vi "шкала вакуума.vi"(11 "Vak_in":dbl) -> (0 "Vak_out_txt":string, 3 "Vak_out":dbl)   [LabVIEW 2016, in "Library.lvlib"]
uses:
  Granule-2000AT/PC/Library.lvlib
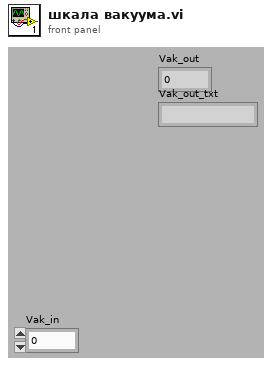
[diagram p1: front panel]
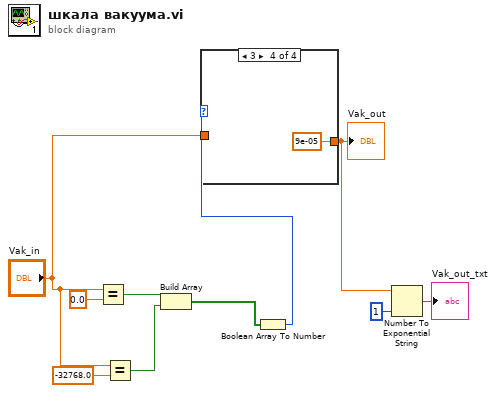
[diagram p0: block diagram]
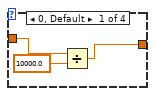
[diagram p2: hidden frame]
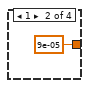
[diagram p3: hidden frame]
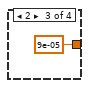
[diagram p4: hidden frame]
diagram:
  n1 = Equal?(x="Vak_in", y=0.0) -> (x = y?=w8:bool)
  n2 = Equal?(x="Vak_in", y=-32768.0) -> (x = y?=w7:bool)
  n3 = Build Array(w8, w7) -> (w6:bool[])
  n4 = Boolean Array To Number(Boolean array=w6) -> (number=w5:u32)
  n5 = case shown="3" w5 {
    tunnel: "Vak_in" -> [w13 _ _ _]
    tunnel: [w11 9e-05 9e-05 9e-05] -> w3
    frame 0, Default {
      n6 = Divide(x=w13, y=10000.0) -> (x/y=w11:dbl)
    }
    frame 1 {
    }
    frame 2 {
    }
    frame 3 {
    }
  }
  "Vak_out" <- w3
  n7 = Number To Exponential String(number=w3, precision (6)=i16 1) -> (E-format string=→"Vak_out_txt":string)  [unwired: 2 in]
